vi "Generador de numeros Sub(vI).vi"() -> (3 "Numeric":i32)   [LabVIEW 2011]
uses:
  <vilib>/express/express arith-compare/Formula/XNode/ExpressFormulaBlockNode.xnode
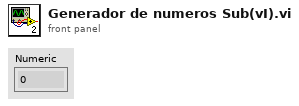
[diagram p1: front panel]
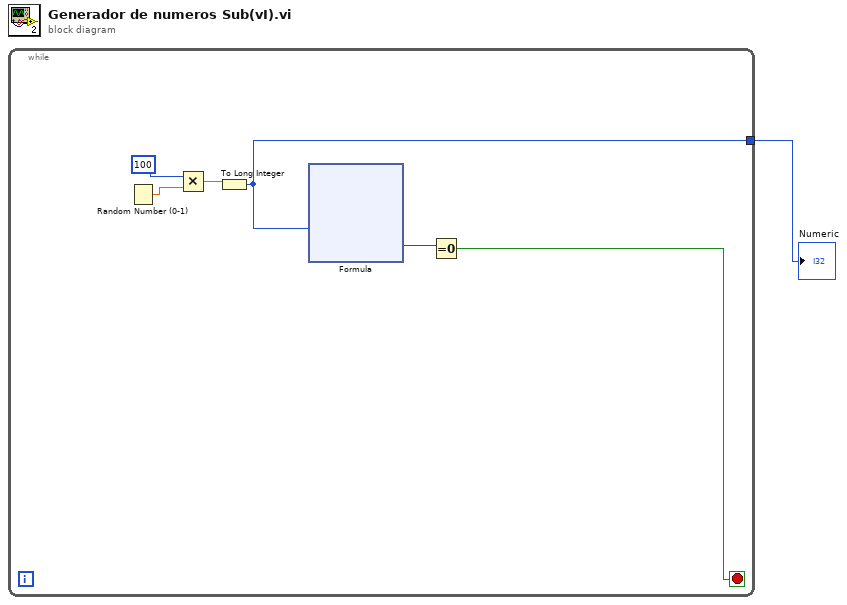
[diagram p0: block diagram]
diagram:
  n1 = while {
    tunnel: [w2] -> w1
    stop <- w3 stop-if-true
    n2 = Random Number (0-1)() -> (number: 0 to 1=w6:dbl)
    n3 = Multiply(x=100, y=w6) -> (x*y=w5:dbl)
    n4 = To Long Integer(number=w5) -> (32bit integer=w2:i32)
    n5 = xnode "Formula"("X1"=w2) -> ("Result"=w4:i32)  [unwired: 1 in, 1 out]
    n6 = Equal To 0?(x=w4) -> (x = 0?=w3:bool)
  }
  "Numeric" <- w1
